vi "USB4000_ACQ.vi"(7 "Type":T1, 8 "error in (no error)":errorcluster, 10 "SpectrumSat":refnum<vi>, 11 "Instruments in":refnum<class "Instruments.lvclass">) -> (0 "error out":errorcluster, 2 "Peak Wl":dbl, 3 "Instruments out":refnum<class "Instruments.lvclass">, 4 "Remeasure":bool)   [LabVIEW 2012, in "Instruments.lvclass"]
uses:
  Instruments.lvclass
  Controls/SpectrometerOphirSelector.ctl
  Instruments.lvclass/Instruments.ctl
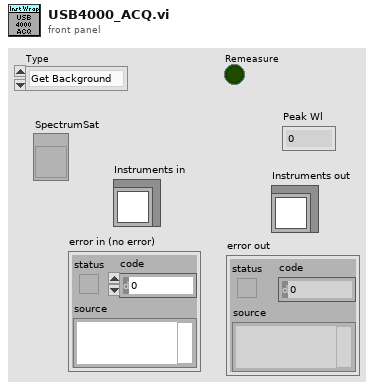
[diagram p1: front panel]
types:
  T1 = typedef "SpectrometerOphirSelector.ctl" = enum16{"Get Background", "Measure", "Measure50", "Raw"}
  T2 = typedef "USB4000_Data.ctl" = cluster{"Wrapper Out":u32, "Number of Spectrometers":i32, "Wavelength":dbl[], "EL Spectrum":dbl[], "Int Time (usec)":i32, bool, "Background":dbl[]}
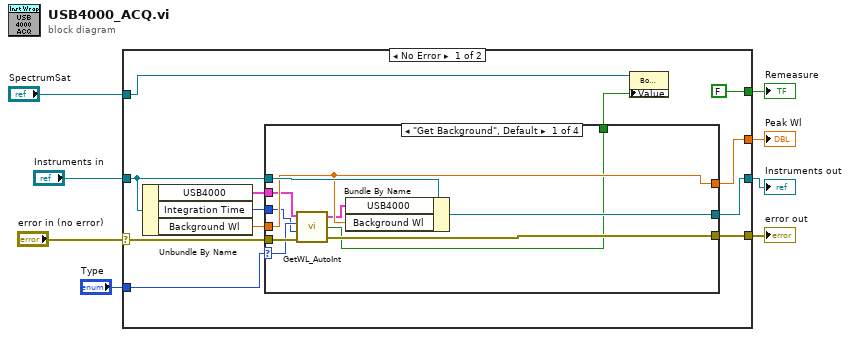
[diagram p0: block diagram]
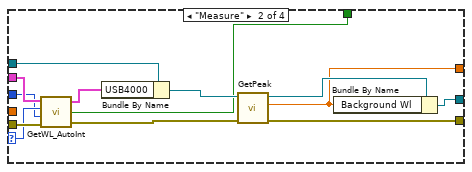
[diagram p2: hidden frame]
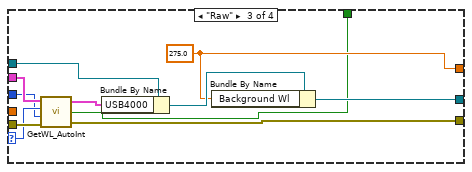
[diagram p3: hidden frame]
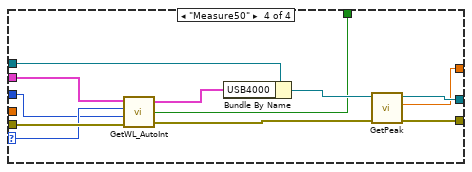
[diagram p4: hidden frame]
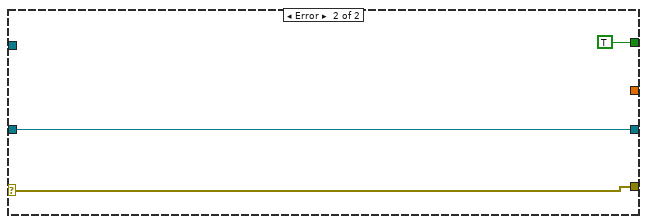
[diagram p5: hidden frame]
diagram:
  n1 = case shown="No Error" "error in (no error)" {
    selector: "error in (no error)" -> [w16 w69]
    tunnel: [w17 w69] -> w7
    tunnel: [w18 w68] -> w5
    tunnel: "Instruments in" -> [w19 w68]
    tunnel: "Type" -> [w13 _]
    tunnel: [w20 _] -> w2
    tunnel: [FALSE TRUE] -> w3
    tunnel: "SpectrumSat" -> [w10 _]
    frame No Error {
      n2 = Unbundle By Name(w19) -> ("USB4000"=w11:T2, "Integration Time"=w15:i32, "Background Wl"=w14:dbl)
      n3 = case shown="\"Get Background\", Default" w13 {
        selector: w13 -> [w23 w33 w47 w57]
        tunnel: w11 -> [w27 w37 w50 w60]
        tunnel: w16 -> [w26 w36 w48 w61]
        tunnel: w19 -> [w30 w43 w54 w65]
        tunnel: [w29 w38 w52 w64] -> w18
        tunnel: [w24 w41 w46 w62] -> w17
        tunnel: [w28 w39 w51 w63] -> w20
        tunnel: w15 -> [w22 w32 w45 w56]
        tunnel: w14 -> [w28 _ _ _]
        tunnel: [w21 w31 w44 w55] -> w9
        frame "Get Background", Default {
          n4 = call "GetWL_AutoInt.vi"("error in (no error)"=w26, "Integration Time"=w22, "Type"=w23, "USB4000 Params In"=w27) -> ("error out"=w24:errorcluster, "Saturated"=w21:bool, "USB4000 Params Out"=w25:T2)
          n5 = Bundle By Name(cluster=w30, "USB4000"=w25, "Background Wl"=w28) -> (w29:refnum<class "Instruments.lvclass">)
        }
        frame "Measure" {
          n6 = call "GetWL_AutoInt.vi"("error in (no error)"=w36, "Integration Time"=w32, "Type"=w33, "USB4000 Params In"=w37) -> ("error out"=w34:errorcluster, "Saturated"=w31:bool, "USB4000 Params Out"=w35:T2)
          n7 = Bundle By Name(cluster=w43, "USB4000"=w35) -> (w42:refnum<class "Instruments.lvclass">)
          n8 = call-dynamic "GetPeak.vi"("error in (no error)"=w34, "Instruments in"=w42) -> ("error out"=w41:errorcluster, "Peak Wl"=w39:dbl, "Instruments out"=w40:refnum<class "Instruments.lvclass">)  [unwired: 7 in]
          n9 = Bundle By Name(cluster=w40, "Background Wl"=w39) -> (w38:refnum<class "Instruments.lvclass">)
        }
        frame "Raw" {
          w51 = 275.0 ("Peak Wl")
          n10 = call "GetWL_AutoInt.vi"("error in (no error)"=w48, "Integration Time"=w45, "Type"=w47, "USB4000 Params In"=w50) -> ("error out"=w46:errorcluster, "Saturated"=w44:bool, "USB4000 Params Out"=w49:T2)
          n11 = Bundle By Name(cluster=w54, "USB4000"=w49) -> (w53:refnum<class "Instruments.lvclass">)
          n12 = Bundle By Name(cluster=w53, "Background Wl"=w51) -> (w52:refnum<class "Instruments.lvclass">)
        }
        frame "Measure50" {
          n13 = call "GetWL_AutoInt.vi"("error in (no error)"=w61, "Integration Time"=w56, "Type"=w57, "USB4000 Params In"=w60) -> ("error out"=w58:errorcluster, "Saturated"=w55:bool, "USB4000 Params Out"=w59:T2)
          n14 = Bundle By Name(cluster=w65, "USB4000"=w59) -> (w66:refnum<class "Instruments.lvclass">)
          n15 = call-dynamic "GetPeak.vi"("error in (no error)"=w58, "Instruments in"=w66) -> ("error out"=w62:errorcluster, "Peak Wl"=w63:dbl, "Instruments out"=w64:refnum<class "Instruments.lvclass">)  [unwired: 7 in]
        }
      }
      n16 = property class="Bool (strict)"(reference=w10, "Value"=w9) -> ()  [unwired: 1 in, 2 out]
    }
    frame Error {
    }
  }
  "error out" <- w7
  "Instruments out" <- w5
  "Peak Wl" <- w2
  "Remeasure" <- w3
